vi "Sample UI.vi"() -> ()   [LabVIEW 2014]
uses:
  Controls/Cron String - STYP.ctl
  Controls/Source Code Control Selection - STYP.ctl
panel:
  out "Build":bool
  in  "Tab Control":enum32{"Information", "Result Text"}(tab)
  in  "Build Type Tab":enum32{"LabVIEW Build", "Blank"}(tab)
  in  "Title 2":string="LabVIEW Build"
  in  "Project Path":path=path "C:/Projects/LabVIEW Continuous Integration/LabVIEW Continuous Integration.lvproj"
  in  "Build Spec":string="Test LabVIEW Launcher"
  in  "Source Code Poll":T1
  in  "Build Trigger":T2={"Day of Week"=enum."Everyday", "Hour"=23, "Enable?"=TRUE} {"Hour" min=0 max=23}
  in  "Jenkins Hostname":string="10.211.55.18:8080"
  in  "Project Name":string="LabVIEW Test"
  in  "How many days to Artifact?":i32=15
  in  "Notification (Separate by Space)":string="brandyn.adderley@ni.com"
  in  "Build Steps(1)":i32(listbox)
  out "Add":bool
  out "Remove":bool
  in  "Step Type":u16(ring) items=["<None>", "LabVIEW Build"]
  in  "Build Text":string
  out "Progress":u8(slide) scale=0.0..100.0
  in  "Title":string="Continuous Integration Project"
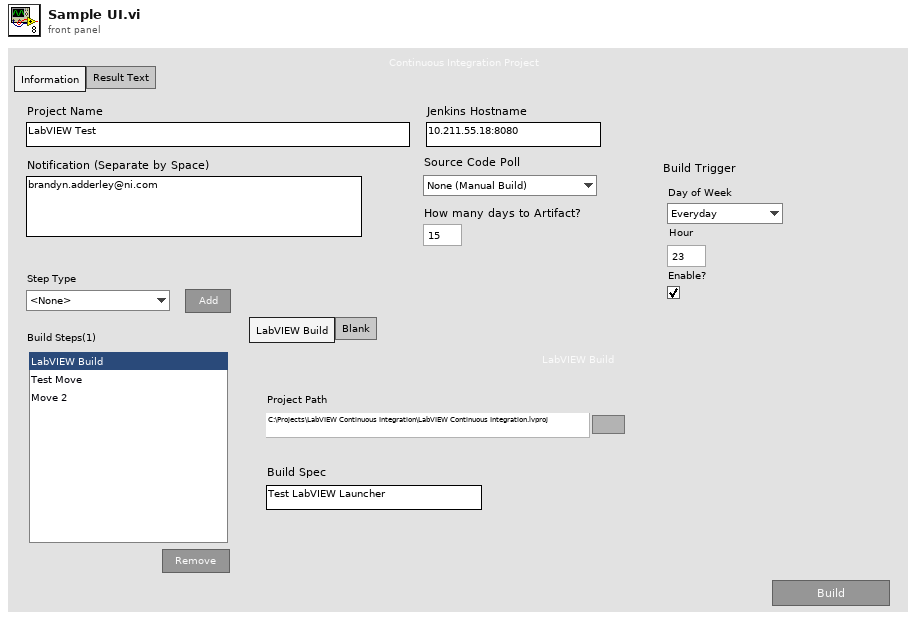
[diagram p1: front panel]
types:
  T1 = typedef "Source Code Control Selection - STYP.ctl" = enum16{"None (Manual Build)", "Every 15 Minutes", "Every 30 Minutes", "Every 45 Minutes", "Every Hour", "Every 2 Hours", "Everyday "}
  T2 = typedef "Cron String - STYP.ctl" = cluster{"Day of Week":enum16{"Everyday", "Sunday", "Monday", "Tuesday", "Wednesday", "Thursday", "Friday", "Saturday"}, "Hour":i32, "Enable?":bool}
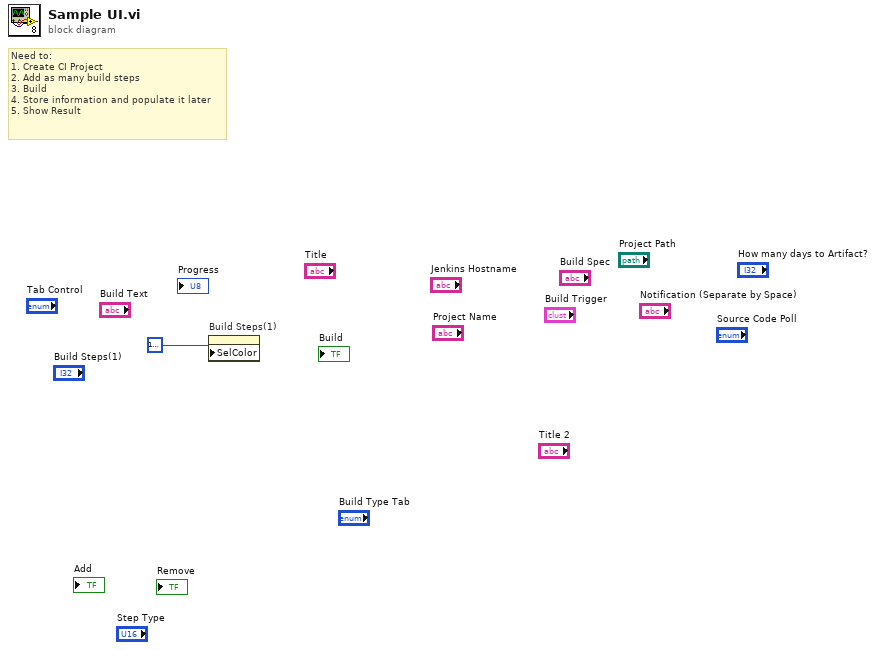
[diagram p0: block diagram]
diagram:
  # "Need to:\n1. Create CI Project\n2. Add as many build steps\n3. Build\n4. Store information and populate it later\n5. Show Result"
  n1 = property on="Build Steps(1)" class="LstBox (strict)"("SelColor"=u32 16777224) -> ()  [unwired: 2 in, 2 out]
